vi "Problem 4.vi"() -> ()   [LabVIEW 2025]
uses:
  fd884f92-0dfc-4c4b-a0db-d76a2bd7cf55.vi
  d81cca8b-5425-422c-848f-b5057428f21b.vi
panel:
  out "Numbers that make palindrome (has duplicates!)":string[](array[string])
  out "Largest 3 Digit Panlidomic Product":i32
  out "List of 3 Digit Palindrom Products":i32[](array[numeric])
  out "Numbers that make palindrome (has duplicates!)":string[](array[string])
  out "List of 2 digit Palindrome Products":i32[](array[numeric])
  out "Largest 2 Digit Panlidomic Product":i32
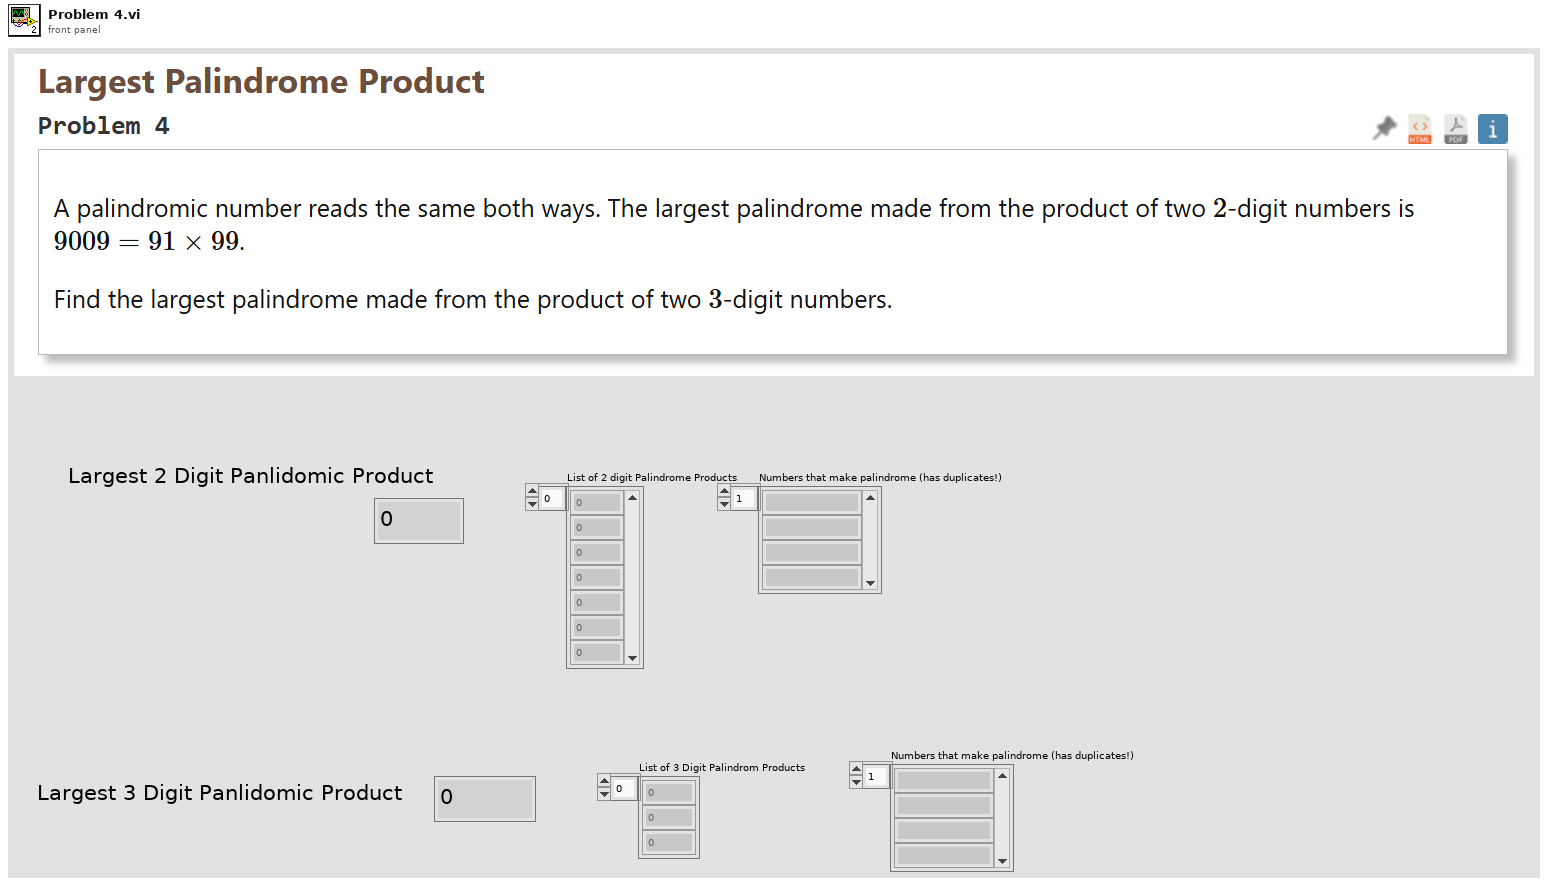
[diagram p1: front panel]
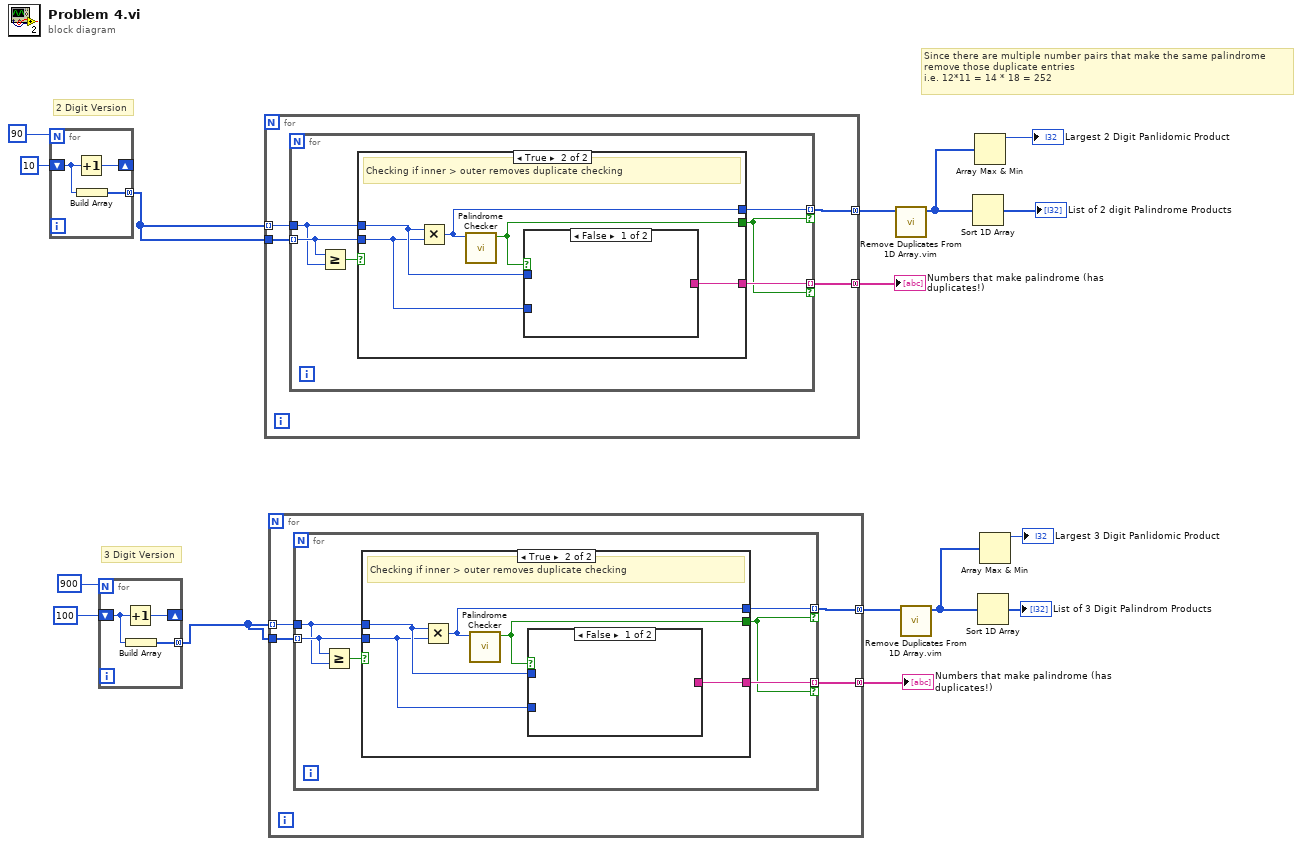
[diagram p0: block diagram]
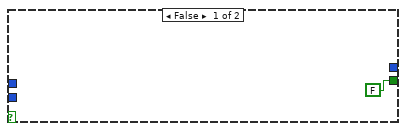
[diagram p2: hidden frame]
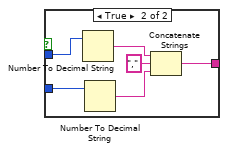
[diagram p3: hidden frame]
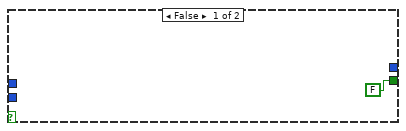
[diagram p4: hidden frame]
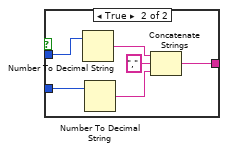
[diagram p5: hidden frame]
diagram:
  # "3 Digit Version"
  # "2 Digit Version"
  # "Since there are multiple number pairs that make the same palindrome\nremove those duplicate entries \ni.e. 12*11 = 14 * 18 = 252"
  n1 = for {
    N: 90 -> [_]
    tunnel: [w19] -> w8 mode=concatenating
    shift-right: [w17] -> _
    shift-left: 10 -> [w18]
    n2 = Increment(x=w18) -> (x+1=w17:i32)
    n3 = Build Array(w18) -> (w19:i32[])
  }
  n4 = for {
    N: 900 -> [_]
    tunnel: [w22] -> w14 mode=concatenating
    shift-right: [w20] -> _
    shift-left: 100 -> [w21]
    n5 = Increment(x=w21) -> (x+1=w20:i32)
    n6 = Build Array(w21) -> (w22:i32[])
  }
  n7 = for {
    tunnel: w8 -> [w25] mode=indexing
    tunnel: w8 -> [w26]
    tunnel: [w24] -> w5 mode=concatenating
    tunnel: [w23] -> w3 mode=concatenating
    n8 = for {
      tunnel: w25 -> [w27]
      tunnel: w26 -> [w28] mode=indexing
      tunnel: [w32] -> w24 mode=indexing if=w31
      tunnel: [w30] -> w23 mode=indexing if=w31
      n9 = Greater Or Equal?(x=w28, y=w27) -> (x >= y?=w29:bool)
      n10 = case shown="True" w29 {
        tunnel: [_ w38] -> w32
        tunnel: [FALSE ("Is Palindromic Number") w34] -> w31
        tunnel: [_ w37] -> w30
        tunnel: w27 -> [_ w36]
        tunnel: w28 -> [_ w35]
        frame False {
        }
        frame True {
          # "Checking if inner > outer removes duplicate checking"
          n11 = Multiply(x=w36, y=w35) -> (x*y=w37:i32)
          n12 = call "Palindrome Checker.vi"("Numeric"=w37) -> ("Is Palindromic Number"=w34:bool)  [unwired: 10 in]
          n13 = case shown="False" w34 {
            tunnel: [_ w44] -> w38
            tunnel: w36 -> [_ w40]
            tunnel: w35 -> [_ w39]
            frame False {
            }
            frame True {
              n14 = Number To Decimal String(number=w40) -> (decimal integer string=w43:string)  [unwired: 1 in]
              n15 = Number To Decimal String(number=w39) -> (decimal integer string=w41:string)  [unwired: 1 in]
              n16 = Concatenate Strings(w43, "," ("string"), w41) -> (w44:string)
            }
          }
        }
      }
    }
  }
  "Numbers that make palindrome (has duplicates!)" <- w5
  n17 = for {
    tunnel: w14 -> [w47] mode=indexing
    tunnel: w14 -> [w48]
    tunnel: [w46] -> w1 mode=concatenating
    tunnel: [w45] -> w12 mode=concatenating
    n18 = for {
      tunnel: w47 -> [w49]
      tunnel: w48 -> [w50] mode=indexing
      tunnel: [w54] -> w46 mode=indexing if=w53
      tunnel: [w52] -> w45 mode=indexing if=w53
      n19 = Greater Or Equal?(x=w50, y=w49) -> (x >= y?=w51:bool)
      n20 = case shown="True" w51 {
        tunnel: [_ w60] -> w54
        tunnel: [FALSE ("Is Palindromic Number") w56] -> w53
        tunnel: [_ w59] -> w52
        tunnel: w49 -> [_ w58]
        tunnel: w50 -> [_ w57]
        frame False {
        }
        frame True {
          # "Checking if inner > outer removes duplicate checking"
          n21 = Multiply(x=w58, y=w57) -> (x*y=w59:i32)
          n22 = call "Palindrome Checker.vi"("Numeric"=w59) -> ("Is Palindromic Number"=w56:bool)  [unwired: 10 in]
          n23 = case shown="False" w56 {
            tunnel: [_ w66] -> w60
            tunnel: w58 -> [_ w62]
            tunnel: w57 -> [_ w61]
            frame False {
            }
            frame True {
              n24 = Number To Decimal String(number=w62) -> (decimal integer string=w65:string)  [unwired: 1 in]
              n25 = Number To Decimal String(number=w61) -> (decimal integer string=w63:string)  [unwired: 1 in]
              n26 = Concatenate Strings(w65, "," ("string"), w63) -> (w66:string)
            }
          }
        }
      }
    }
  }
  "Numbers that make palindrome (has duplicates!)" <- w1
  n27 = call "Remove Duplicates From 1D Array.vim"("array"=w3) -> ("array with duplicates removed"=w2:i32[])  [unwired: 10 in]
  n28 = call "Remove Duplicates From 1D Array.vim"("array"=w12) -> ("array with duplicates removed"=w13:i32[])  [unwired: 10 in]
  n29 = Sort 1D Array(array=w2) -> (sorted array=→"List of 2 digit Palindrome Products":i32[])
  n30 = Array Max & Min(array=w2) -> (max value=→"Largest 2 Digit Panlidomic Product":i32)  [unwired: 3 out]
  n31 = Sort 1D Array(array=w13) -> (sorted array=→"List of 3 Digit Palindrom Products":i32[])
  n32 = Array Max & Min(array=w13) -> (max value=→"Largest 3 Digit Panlidomic Product":i32)  [unwired: 3 out]
